vi "Bild_aufhellen_bzw_verdunkeln.vi"(6 "Y-Min":i32, 7 "X-Min":i32, 9 "Y-Max":i32, 10 "X-Max":i32, 11 "Image Pixels (U8) in":u8[][](array[numeric])) -> (3 "Image Pixels (U8) out":u8[][](array[numeric]))   [LabVIEW 2014]
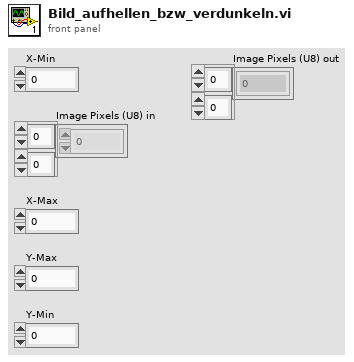
[diagram p1: front panel]
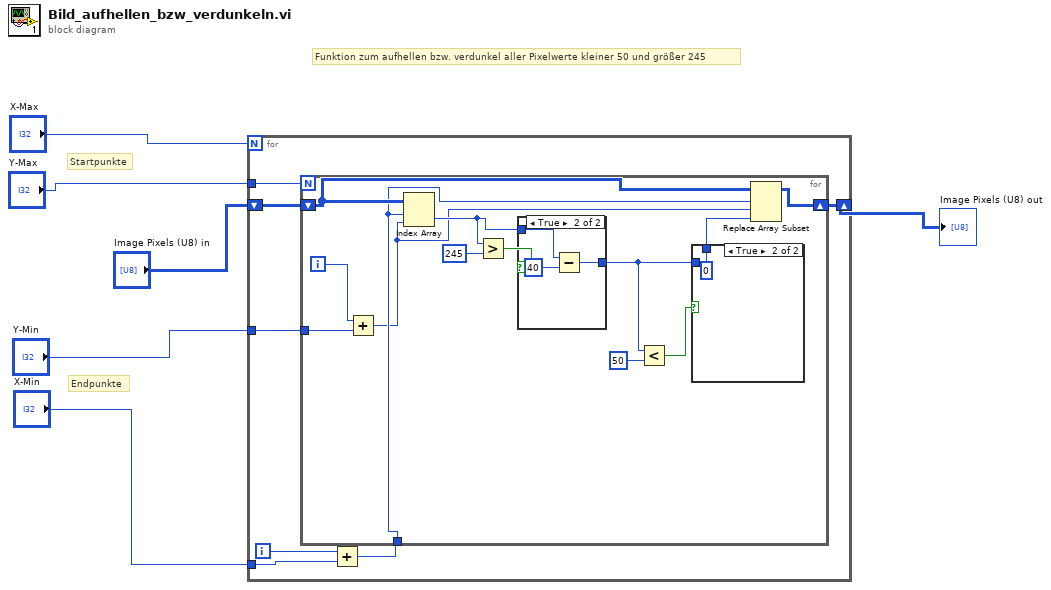
[diagram p0: block diagram]
diagram:
  # "Endpunkte"
  # "Startpunkte"
  # "Funktion zum aufhellen bzw. verdunkel aller Pixelwerte kleiner 50 und größer 245"
  n1 = for {
    N: "X-Max" -> [_]
    shift-right: [w12] -> w3
    shift-left: "Image Pixels (U8) in" -> [w13]
    tunnel: "Y-Max" -> [w9]
    tunnel: "Y-Min" -> [w8]
    tunnel: "X-Min" -> [w7]
    i -> [w11]
    n2 = Add(x=w11, y=w7) -> (x+y=w10:i32)
    n3 = for {
      N: w9 -> [_]
      shift-right: [w25] -> w12
      shift-left: w13 -> [w26]
      tunnel: w10 -> [w24]
      tunnel: w8 -> [w15]
      i -> [w16]
      n4 = Add(x=w16, y=w15) -> (x+y=w14:i32)
      n5 = Index Array(array=w26, index (row)=w24, index (col)=w14) -> (element=w21:u8)
      n6 = Greater?(x=w21, y=u8 245) -> (0:w22:bool)
      n7 = case shown="True" w22 {
        tunnel: w21 -> [w29 w32]
        tunnel: [w29 w30] -> w19
        frame False {
        }
        frame True {
          n8 = Subtract(x=w32, y=u8 40) -> (x-y=w30:u8)
        }
      }
      n9 = Less?(x=w19, y=u8 50) -> (x < y?=w18:bool)
      n10 = case shown="True" w18 {
        tunnel: w19 -> [w27 _]
        tunnel: [w27 u8 0] -> w17
        frame False {
        }
        frame True {
        }
      }
      n11 = Replace Array Subset(array=w26, new element=w17, index (row)=w24, index (col)=w14) -> (w25:u8[][])
    }
  }
  "Image Pixels (U8) out" <- w3
